vi "Read_MNK_B_Field.vi"(8 "Read from DSC in":errorcluster) -> (0 "Read from DSC":errorcluster, 1 "Field Rate":dbl, 2 "Field":dbl)   [LabVIEW 2016, in "Instrument.OxfordVRM.lvclass"]
uses:
  Instrument.OxfordVRM.lvclass
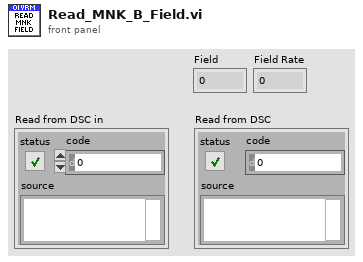
[diagram p1: front panel]
types:
  T1 = typedef "Instrument.OxfordVRM.lvclass/Status.ctl" = cluster{"Magnet Field":dbl, "PS Field":dbl, "Target Field":dbl, "Target Field Rate":dbl, "Voltage":dbl, "Current":dbl, "Switch":bool, "Mercury State":string}
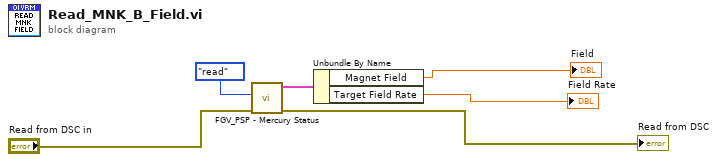
[diagram p0: block diagram]
diagram:
  n1 = call "FGV_PSP - Mercury Status.vi"("error in"="Read from DSC in", "Function"=enum16{"write", "read"}."read") -> ("error out"=→"Read from DSC":errorcluster, "Status"=w6:T1)  [unwired: 4 in]
  n2 = Unbundle By Name(w6) -> ("Magnet Field"=→"Field":dbl, "Target Field Rate"=→"Field Rate":dbl)
